vi "read channel limits config.vi"(10 "config data in":T19={"Message"={"Parameters"={"FPGA Ref"=refnum, "configID"=0, "activeChannels"=[]}, "Variables"={"RT Status"={"Comms loop"=FALSE, "scheduler loop"=FALSE, "data process loop"=FALSE, "FIFO loop"=FALSE, "Command Stream"=FALSE, "Error Stream"=FALSE, "FPGA FIFO"=FALSE, "Data Stream"=FALSE}, "watchdog"=timestamp(0 s since 1904-01-01), "limitsEnabled"=FALSE, "Interlocks"={"gearboxOil"=FALSE, "bearingOil"=FALSE, "gearboxAir"=FALSE}}}, "FIFO"={"Params"={"FPGA ref"=refnum, "Total Channels"=0}, "Variables"={"FIFO wait counter"=0, "FIFO read trigger"=0}}, "Comms data"={"Parameters"={"error writer name"="", "command reader name"="", "error buffer size"=0, "command buffer size"=0, "scanivalveIP"="", "scanivalvePeriod"=0}, "Variables"={"listen schedule"=0, "incident buffer"=[], "command stream"="", "error stream"="", "waiting for command stream connect"=FALSE, "waiting for error stream connect"=FALSE, "scanivalve connection"=refnum, "scanivalveScheduleID"=0, "activeScanivalvePorts"=[], "channelCount"=0}, "scanivalveConfig"={"listS"={"period"=0, "ADtrig"=FALSE, "ScanTrig"=FALSE, "page"=0, "qpkts"=0}, "listC"={"ZC"=FALSE, "unitScan"="", "CvtUnit"=0.0, "bin"=FALSE, "EU"=FALSE}, "listSG"={"Avg1"=0, "FPS1"=0, "SGEnable1"=FALSE}, "activeChannels"={"Chan1"={"101"=FALSE, "102"=FALSE, "103"=FALSE, "104"=FALSE, "109"=FALSE, "110"=FALSE, "111"=FALSE, "112"=FALSE, "201"=FALSE, "202"=FALSE, "203"=FALSE, "204"=FALSE, "209"=FALSE, "210"=FALSE, "211"=FALSE, "212"=FALSE, "301"=FALSE, "302"=FALSE, "303"=FALSE, "304"=FALSE, "309"=FALSE, "310"=FALSE, "311"=FALSE, "312"=FALSE, "401"=FALSE, "402"=FALSE, "403"=FALSE, "404"=FALSE, "409"=FALSE, "410"=FALSE, "411"=FALSE, "412"=FALSE}}}}, "Data processor"={"Parameters"={"FPGA Ref"=refnum, "data stream"={"data writer name"="error writer", "NS write buffer size"=16, "NS Buffer length"=0}, "FIFO Depth"=0, "Channel controls"={"FIFO channel count"=0, "active indices"=[], "active channels"=0, "channelScaling"=[], "scanivalveCount"=0, "channels"=[]}, "safetyChannels"={"oilP"=0, "airP"=0, "water"=0, "channelLimits"=[]}, "speedChannel"=0, "maxSpeedLimit"=0.0, "Torque"={"fixedOffset"=0.0, "filter"=FALSE, "fallingEdge"=FALSE, "swapEncoders"=FALSE}}, "Variables"={"Intermediary buffer"=[], "buffer position"=0, "write loop counter"=0, "NS write trigger"=0, "NS Connection status"=FALSE, "waiting for NS"=FALSE, "labAmbient"={"pressure"=0.0, "temperature"=0.0}, "scanivalvePorts"=[], "scanivalvePressures"=[], "data stream"="", "activeChannelLimitIndex"=[], "runningSpeedLimit"=0.0, "speedChannelIndex"=0, "Interlocks"={"gearboxOil"=FALSE, "bearingOil"=FALSE, "gearboxAir"=FALSE}, "interlockChannels"={"gearboxOil"=0, "bearingOil"=0, "air"=0}, "limitStates"=[]}}}, 11 "configFile ref":T1) -> (3 "config data out":T19={"Message"={"Parameters"={"FPGA Ref"=refnum, "configID"=0, "activeChannels"=[]}, "Variables"={"RT Status"={"Comms loop"=FALSE, "scheduler loop"=FALSE, "data process loop"=FALSE, "FIFO loop"=FALSE, "Command Stream"=FALSE, "Error Stream"=FALSE, "FPGA FIFO"=FALSE, "Data Stream"=FALSE}, "watchdog"=timestamp(0 s since 1904-01-01), "limitsEnabled"=FALSE, "Interlocks"={"gearboxOil"=FALSE, "bearingOil"=FALSE, "gearboxAir"=FALSE}}}, "FIFO"={"Params"={"FPGA ref"=refnum, "Total Channels"=0}, "Variables"={"FIFO wait counter"=0, "FIFO read trigger"=0}}, "Comms data"={"Parameters"={"error writer name"="", "command reader name"="", "error buffer size"=0, "command buffer size"=0, "scanivalveIP"="", "scanivalvePeriod"=0}, "Variables"={"listen schedule"=0, "incident buffer"=[], "command stream"="", "error stream"="", "waiting for command stream connect"=FALSE, "waiting for error stream connect"=FALSE, "scanivalve connection"=refnum, "scanivalveScheduleID"=0, "activeScanivalvePorts"=[], "channelCount"=0}, "scanivalveConfig"={"listS"={"period"=0, "ADtrig"=FALSE, "ScanTrig"=FALSE, "page"=0, "qpkts"=0}, "listC"={"ZC"=FALSE, "unitScan"="", "CvtUnit"=0.0, "bin"=FALSE, "EU"=FALSE}, "listSG"={"Avg1"=0, "FPS1"=0, "SGEnable1"=FALSE}, "activeChannels"={"Chan1"={"101"=FALSE, "102"=FALSE, "103"=FALSE, "104"=FALSE, "109"=FALSE, "110"=FALSE, "111"=FALSE, "112"=FALSE, "201"=FALSE, "202"=FALSE, "203"=FALSE, "204"=FALSE, "209"=FALSE, "210"=FALSE, "211"=FALSE, "212"=FALSE, "301"=FALSE, "302"=FALSE, "303"=FALSE, "304"=FALSE, "309"=FALSE, "310"=FALSE, "311"=FALSE, "312"=FALSE, "401"=FALSE, "402"=FALSE, "403"=FALSE, "404"=FALSE, "409"=FALSE, "410"=FALSE, "411"=FALSE, "412"=FALSE}}}}, "Data processor"={"Parameters"={"FPGA Ref"=refnum, "data stream"={"data writer name"="error writer", "NS write buffer size"=16, "NS Buffer length"=0}, "FIFO Depth"=0, "Channel controls"={"FIFO channel count"=0, "active indices"=[], "active channels"=0, "channelScaling"=[], "scanivalveCount"=0, "channels"=[]}, "safetyChannels"={"oilP"=0, "airP"=0, "water"=0, "channelLimits"=[]}, "speedChannel"=0, "maxSpeedLimit"=0.0, "Torque"={"fixedOffset"=0.0, "filter"=FALSE, "fallingEdge"=FALSE, "swapEncoders"=FALSE}}, "Variables"={"Intermediary buffer"=[], "buffer position"=0, "write loop counter"=0, "NS write trigger"=0, "NS Connection status"=FALSE, "waiting for NS"=FALSE, "labAmbient"={"pressure"=0.0, "temperature"=0.0}, "scanivalvePorts"=[], "scanivalvePressures"=[], "data stream"="", "activeChannelLimitIndex"=[], "runningSpeedLimit"=0.0, "speedChannelIndex"=0, "Interlocks"={"gearboxOil"=FALSE, "bearingOil"=FALSE, "gearboxAir"=FALSE}, "interlockChannels"={"gearboxOil"=0, "bearingOil"=0, "air"=0}, "limitStates"=[]}}})   [LabVIEW 2018]
uses:
  Type Defs/Message loop data.ctl
  Type Defs/FPGA reference.ctl
  Type Defs/RT Status.ctl
  Type Defs/Analogue loop data.ctl
  Communications loop/comms data.ctl
  Type Defs/generic incident.ctl
  ICL-LabVIEW_General/Scanivalve API project/full interface/polymorphic/scanivalveConfig.ctl
  ICL-LabVIEW_General/Scanivalve API project/full interface/listS.ctl
  ICL-LabVIEW_General/Scanivalve API project/full interface/listC.ctl
  ICL-LabVIEW_General/Scanivalve API project/full interface/listSG.ctl
  ICL-LabVIEW_General/Scanivalve API project/full interface/chan1.ctl
  Type Defs/Data processing loop data.ctl
  PC/type defs/channelControl.ctl
  Type Defs/channelScalingTypes.ctl
  Type Defs/scalingMethods.ctl
  ICL-LabVIEW_General/data channels/parent class/Data Channel.lvclass
  PC/type defs/channelLimitControl.ctl
  PC/type defs/limitActions.ctl
  <vilib>/Utility/config.llb/Config Data RefNum.ctl
  <vilib>/Utility/config.llb/Read Key (U32).vi
  <vilib>/Utility/config.llb/Read Key (Boolean).vi
  <vilib>/Utility/config.llb/Read Key (Double).vi
  <vilib>/Utility/config.llb/Read Key (I32).vi
  <vilib>/Utility/config.llb/NI_LVConfig.lvlib
  ICL-LabVIEW_General/Scanivalve API project/Scanivalve API.lvlib
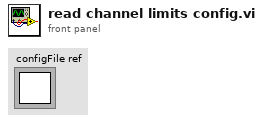
[diagram p1: front panel]
types:
  T1 = typedef "NI_LVConfig.lvlib/Config Data RefNum.ctl" = refnum<k1>
  T2 = typedef "Message loop data.ctl" = cluster{"Parameters":cluster{"FPGA Ref":T3, "configID":u32, "activeChannels":cluster{"index":u16, "name":string}[]}, "Variables":cluster{"RT Status":T4, "watchdog":timestamp, "limitsEnabled":bool, "Interlocks":cluster{"gearboxOil":bool, "bearingOil":bool, "gearboxAir":bool}}}
  T3 = typedef "FPGA reference.ctl" = refnum<k20>
  T4 = typedef "RT Status.ctl" = cluster{"Comms loop":bool, "scheduler loop":bool, "data process loop":bool, "FIFO loop":bool, "Command Stream":bool, "Error Stream":bool, "FPGA FIFO":bool, "Data Stream":bool}
  T5 = typedef "Analogue loop data.ctl" = cluster{"Params":cluster{"FPGA ref":T3, "Total Channels":u32}, "Variables":cluster{"FIFO wait counter":u16, "FIFO read trigger":u32}}
  T6 = typedef "comms data.ctl" = cluster{"Parameters":cluster{"error writer name":string, "command reader name":string, "error buffer size":i32, "command buffer size":i32, "scanivalveIP":string, "scanivalvePeriod":u16}, "Variables":cluster{"listen schedule":u32, "incident buffer":T7[], "command stream":refnum<k21>, "error stream":refnum<k21>, "waiting for command stream connect":bool, "waiting for error stream connect":bool, "scanivalve connection":refnum<k5>, "scanivalveScheduleID":u32, "activeScanivalvePorts":i32[], "channelCount":i16}, "scanivalveConfig":T8}
  T7 = typedef "generic incident.ctl" = cluster{"timestamp":timestamp, "type":string, "Variant":variant}
  T8 = typedef "Scanivalve API.lvlib/scanivalveConfig.ctl" = cluster{"listS":T9, "listC":T10, "listSG":T11, "activeChannels":T12}
  T9 = typedef "Scanivalve API.lvlib/listS.ctl" = cluster{"period":u16, "ADtrig":bool, "ScanTrig":bool, "page":u16, "qpkts":u16}
  T10 = typedef "Scanivalve API.lvlib/listC.ctl" = cluster{"ZC":bool, "unitScan":string, "CvtUnit":dbl, "bin":bool, "EU":bool}
  T11 = typedef "Scanivalve API.lvlib/listSG.ctl" = cluster{"Avg1":u16, "FPS1":u16, "SGEnable1":bool}
  T12 = typedef "Scanivalve API.lvlib/chan1.ctl" = cluster{"Chan1":cluster{"101":bool, "102":bool, "103":bool, "104":bool, "109":bool, "110":bool, "111":bool, "112":bool, "201":bool, "202":bool, "203":bool, "204":bool, "209":bool, "210":bool, "211":bool, "212":bool, "301":bool, "302":bool, "303":bool, "304":bool, "309":bool, "310":bool, "311":bool, "312":bool, "401":bool, "402":bool, "403":bool, "404":bool, "409":bool, "410":bool, "411":bool, "412":bool}}
  T13 = typedef "Data processing loop data.ctl" = cluster{"Parameters":cluster{"FPGA Ref":T3, "data stream":cluster{"data writer name":string, "NS write buffer size":i32, "NS Buffer length":u32}, "FIFO Depth":u32, "Channel controls":cluster{"FIFO channel count":i32, "active indices":i16[], "active channels":i32, "channelScaling":T14[], "scanivalveCount":i32, "channels":refnum<class "Data Channel.lvclass">[]}, "safetyChannels":cluster{"oilP":u16, "airP":u16, "water":u16, "channelLimits":T17[]}, "speedChannel":i32, "maxSpeedLimit":dbl, "Torque":cluster{"fixedOffset":dbl, "filter":bool, "fallingEdge":bool, "swapEncoders":bool}}, "Variables":cluster{"Intermediary buffer":dbl[][], "buffer position":u32, "write loop counter":u16, "NS write trigger":u32, "NS Connection status":bool, "waiting for NS":bool, "labAmbient":cluster{"pressure":dbl, "temperature":dbl}, "scanivalvePorts":u16[], "scanivalvePressures":dbl[], "data stream":refnum<k21>, "activeChannelLimitIndex":u16[], "runningSpeedLimit":dbl, "speedChannelIndex":i32, "Interlocks":cluster{"gearboxOil":bool, "bearingOil":bool, "gearboxAir":bool}, "interlockChannels":cluster{"gearboxOil":i32, "bearingOil":i32, "air":i32}, "limitStates":cluster{"warn":bool, "alarm":bool}[]}}
  T14 = typedef "channelControl.ctl" = cluster{"index":u16, "active":bool, "channelType":T15, "module":u16, "terminal":u16, "channelName":string, "scalingMethod":T16, "scalingParameters":dbl[], "scaledUnits":string, "tempOffset":dbl}
  T15 = typedef "channelScalingTypes.ctl" = enum16{"calculation", "measurement", "scanivalve", "output", "digital"}
  T16 = typedef "scalingMethods.ctl" = enum16{"none", "linear", "thermocouple", "polynomial", "encoder", "RTD"}
  T17 = typedef "channelLimitControl.ctl" = cluster{"channelID":u16, "Enabled":bool, "warnValue":dbl, "limitValue":dbl, "Invert":bool, "limitAction":T18}
  T18 = typedef "limitActions.ctl" = enum16{"stop", "shutdown", "ignore"}
  T19 = cluster{"Message":T2, "FIFO":T5, "Comms data":T6, "Data processor":T13}
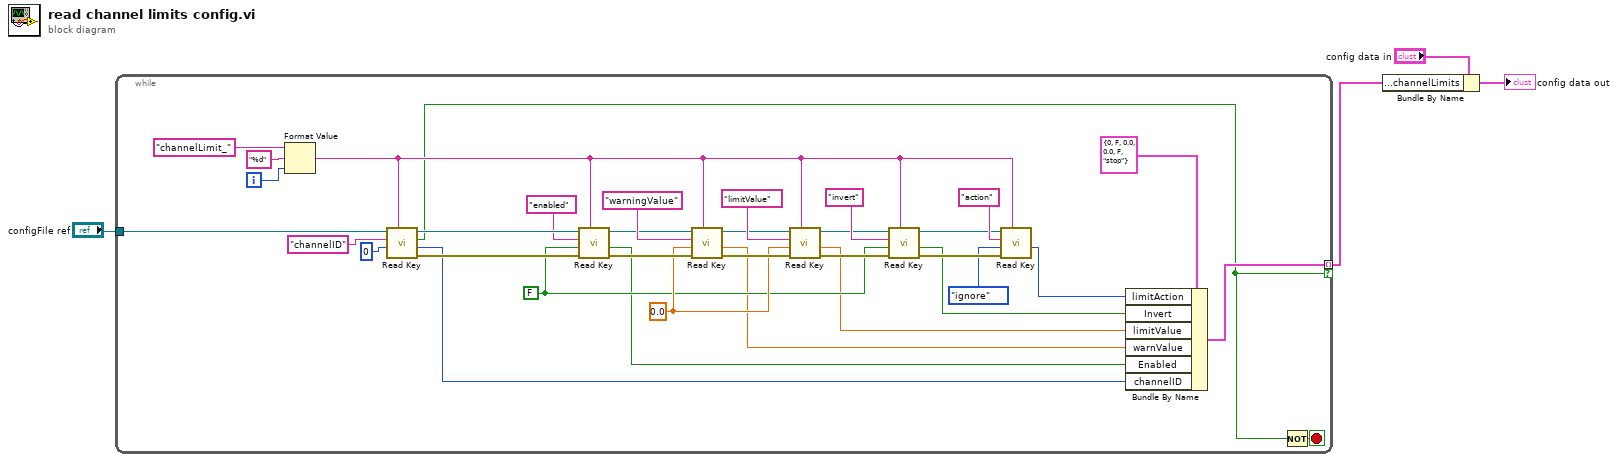
[diagram p0: block diagram]
diagram:
  n1 = while {
    tunnel: "configFile ref" -> [w33]
    tunnel: [w32] -> w1 mode=indexing if=w6
    i -> [w39]
    stop <- w5 stop-if-true
    w14 = 0.0 ("warnValue")
    w13 = FALSE ("default value")
    n2 = Format Value(string ("")="channelLimit_", format string="%d", value (0)=w39) -> (output string=w29:string)
    n3 = call-poly <vilib>:"Read Key.vi"("section"=w29, "default value"=u16 0 ("channelID"), "key"="channelID", "refnum"=w33) -> ("error out"=w35:errorcluster, "value"=w30:u32, "found?"=w6:bool, "refnum out"=w34:T1)  [unwired: 4 in]
    n4 = call-poly <vilib>:"Read Key.vi"("section"=w29, "error in (no error)"=w35, "default value"=w13, "key"="enabled", "refnum"=w34) -> ("error out"=w23:errorcluster, "value"=w11:bool, "refnum out"=w22:T1)  [unwired: 3 in, 1 out]
    n5 = call-poly <vilib>:"Read Key.vi"("section"=w29, "error in (no error)"=w23, "default value"=w14, "key"="warningValue", "refnum"=w22) -> ("error out"=w20:errorcluster, "value"=w10:dbl, "refnum out"=w21:T1)  [unwired: 3 in, 1 out]
    n6 = call-poly <vilib>:"Read Key.vi"("section"=w29, "error in (no error)"=w20, "default value"=w14, "key"="limitValue", "refnum"=w21) -> ("error out"=w19:errorcluster, "value"=w9:dbl, "refnum out"=w18:T1)  [unwired: 3 in, 1 out]
    n7 = call-poly <vilib>:"Read Key.vi"("section"=w29, "error in (no error)"=w19, "default value"=w13, "key"="invert", "refnum"=w18) -> ("error out"=w17:errorcluster, "value"=w8:bool, "refnum out"=w16:T1)  [unwired: 3 in, 1 out]
    n8 = call-poly <vilib>:"Read Key.vi"("section"=w29, "error in (no error)"=w17, "default value"=limitActions."ignore" ("limitAction"), "key"="action", "refnum"=w16) -> ("value"=w7:i32)  [unwired: 3 in, 3 out]
    n9 = Bundle By Name(cluster=T17 {"channelID"=0, "Enabled"=FALSE, "warnValue"=0.0, "limitValue"=0.0, "Invert"=FALSE, "limitAction"=enum."stop"} ("Temperature monitoring"), "limitAction"=w7, "Invert"=w8, "limitValue"=w9, "warnValue"=w10, "Enabled"=w11, "channelID"=w30) -> (w32:T17)
    n10 = Not(x=w6) -> (.not. x?=w5:bool)
  }
  n11 = Bundle By Name(cluster="config data in", "Data processor.Parameters.safetyChannels.channelLimits"=w1) -> (→"config data out":T19)
